vi "load or save device list.vi"(6 "Type":string="Device ", 7 "Mode":u16(ring) items=["Load", "Save"], 10 "selected path":path, 11 "List of devices in":T1 {"List of locations"."Position"."Position Y" format="%#.3f"; "List of locations"."Position"."Position X" format="%#.3f"}) -> (2 "file path out":path, 3 "List of devices out":T1 {"List of locations"."Position"."Position Y" format="%#.3f"; "List of locations"."Position"."Position X" format="%#.3f"})   [LabVIEW 2017]
uses:
  device_list.ctl
  device.ctl
  location.ctl
  <vilib>/Utility/config.llb/Read Key (String).vi
  <vilib>/Utility/config.llb/Write Key (String).vi
  <vilib>/regexp/Match Regular Expression.xnode
  <vilib>/Utility/config.llb/NI_LVConfig.lvlib
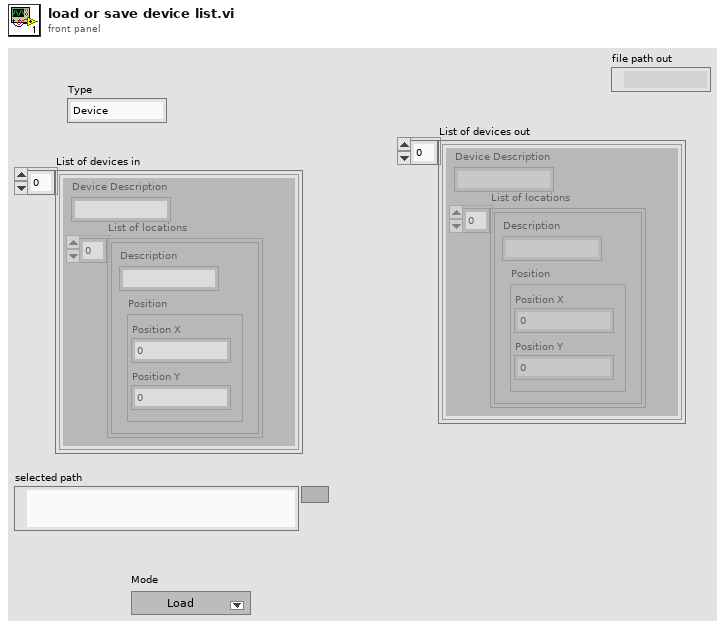
[diagram p1: front panel]
types:
  T1 = typedef "device_list.ctl" = T2[]
  T2 = typedef "device.ctl" = cluster{"List of locations":T3[], "Device Description":string}
  T3 = typedef "location.ctl" = cluster{"Description":string, "Position":cluster{"Position X":dbl, "Position Y":dbl}}
  T4 = typedef "NI_LVConfig.lvlib/Config Data RefNum.ctl" = refnum<k1>
  T5 = cluster{"array type (2D Dbl)[0]":dbl, "array type (2D Dbl)[1]":dbl}
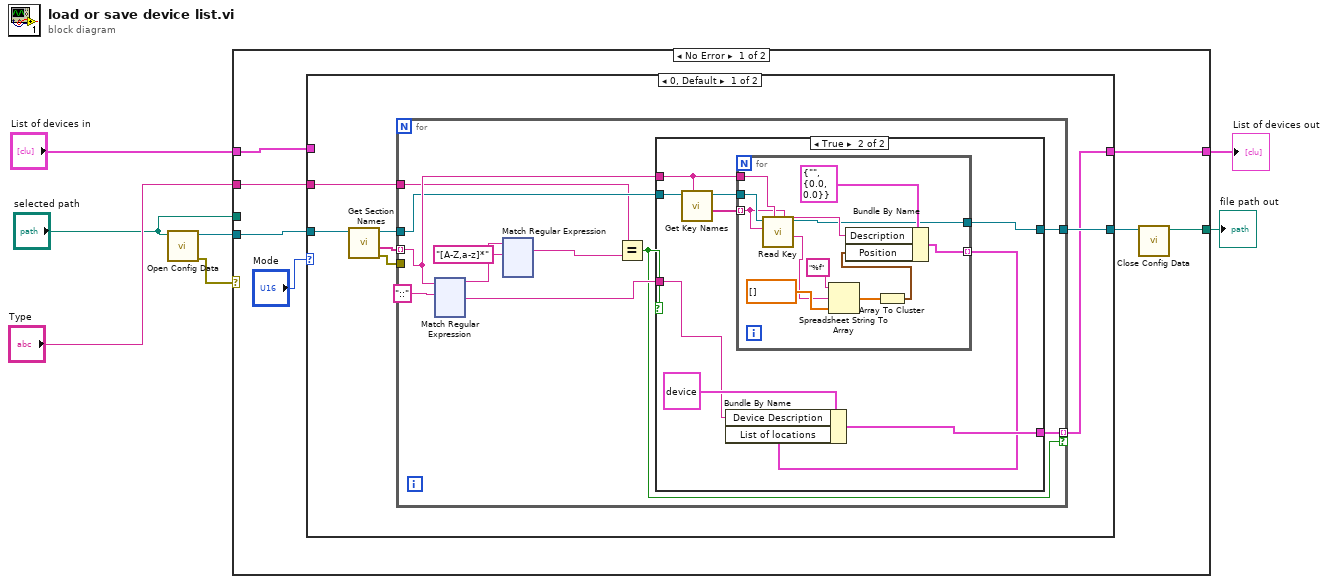
[diagram p0: block diagram]
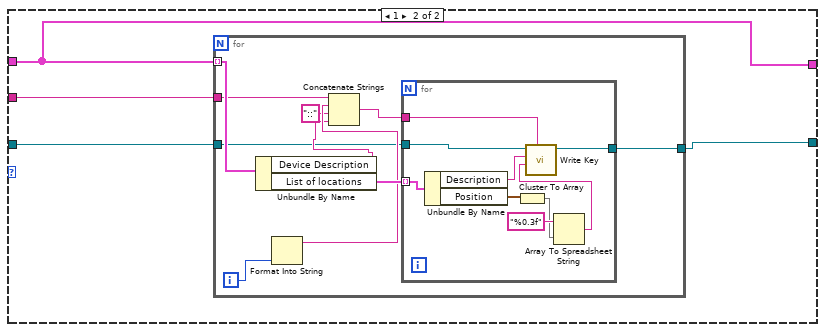
[diagram p3: hidden frame]
diagram:
  n1 = call <vilib>:"Open Config Data.vi"("configuration file path"="selected path") -> ("error out"=w4:errorcluster, "refnum"=w7:T4)  [unwired: 8 in, 1 out]
  n2 = case shown="No Error" w4 {
    tunnel: w7 -> [w14 _]
    tunnel: "List of devices in" -> [w13 w306]
    tunnel: [w10 w306] -> w6
    tunnel: "Type" -> [w9 _]
    tunnel: [w8 w305] -> w2
    tunnel: "selected path" -> [_ w305]
    frame No Error {
      n3 = case shown="0, Default" "Mode" {
        tunnel: w14 -> [w21 w285]
        tunnel: w13 -> [_ w283]
        tunnel: [w18 w284] -> w11
        tunnel: [w17 w283] -> w10
        tunnel: w9 -> [w15 w282]
        frame 0, Default {
          n4 = call <vilib>:"Get Section Names.vi"("refnum"=w21) -> ("error out"=w16:errorcluster, "section names"=w20:string[], "refnum out"=w19:T4)  [unwired: 8 in]
          n5 = for {
            tunnel: w20 -> [w31] mode=indexing
            tunnel: w19 -> [w28]
            tunnel: [w30] -> w18
            tunnel: [w29] -> w17 mode=indexing if=w26
            tunnel: w16 -> [_]
            tunnel: w15 -> [w23]
            n6 = xnode "Match Regular Expression"("input string"=w31, "regular expression"="::") -> ("before match"=w25:string, "after match"=w32:string)  [unwired: 4 in, 3 out]
            n7 = xnode "Match Regular Expression"("input string"=w25, "regular expression"="[A-Z,a-z]*") -> ("whole match"=w22:string)  [unwired: 4 in, 4 out]
            n8 = Equal?(x=w23, y=w22) -> (x = y?=w26:bool)
            n9 = case shown="True" w26 {
              tunnel: w32 -> [_ w154]
              tunnel: w31 -> [_ w152]
              tunnel: [w147 w151] -> w30
              tunnel: [_ w150] -> w29
              tunnel: w28 -> [w147 w149]
              frame False {
              }
              frame True {
                n10 = call <vilib>:"Get Key Names.vi"("section"=w152, "refnum"=w149) -> ("key names"=w156:string[], "refnum out"=w153:T4)  [unwired: 6 in, 2 out]
                n11 = for {
                  tunnel: w156 -> [w162] mode=indexing
                  tunnel: w153 -> [w163]
                  tunnel: w152 -> [w164]
                  tunnel: [w161] -> w151
                  tunnel: [w160] -> w148 mode=indexing
                  n12 = call-poly <vilib>:"Read Key.vi"("section"=w164, "key"=w162, "refnum"=w163) -> ("value"=w158:string, "refnum out"=w161:T4)  [unwired: 5 in, 2 out]
                  n13 = Spreadsheet String To Array(format string="%f", spreadsheet string=w158, array type (2D Dbl)=dbl[] []) -> (array=w165:dbl[])  [unwired: 1 in]
                  n14 = Array To Cluster(array=w165) -> (cluster=w157:T5)
                  n15 = Bundle By Name(cluster=T3 {"Description"="", "Position"={"Position X"=0.0, "Position Y"=0.0}} ("Location"), "Description"=w162, "Position"=w157) -> (w160:T3)
                }
                n16 = Bundle By Name(cluster=T2 {"List of locations"=[{"Description"="Input", "Position"={"Position X"=0.0, "Position Y"=0.0}}, {"Description"="MZI", "Position"={"Position X"=0.0, "Position Y"=10.0}}, {"Description"="Fluid Pool", "Position"={"Position X"=0.0, "Position Y"=20.0}}, {"Description"="Output", "Position"={"Position X"=0.0, "Position Y"=30.0}}], "Device Description"="Default"} ("Defualt Device"), "Device Description"=w154, "List of locations"=w148) -> (w150:T2)
              }
            }
          }
        }
        frame 1 {
          n17 = for {
            tunnel: w283 -> [w295] mode=indexing
            tunnel: w285 -> [w289]
            tunnel: [w288] -> w284
            tunnel: w282 -> [w286]
            i -> [w292]
            n18 = Unbundle By Name(w295) -> ("Device Description"=w290:string, "List of locations"=w294:T3[])
            n19 = Format Into String(w292) -> (resulting string=w291:string)  [unwired: 3 in, 1 out]
            n20 = Concatenate Strings(w286, w291, "::" ("string"), w290) -> (w293:string)
            n21 = for {
              tunnel: w294 -> [w304] mode=indexing
              tunnel: w293 -> [w296]
              tunnel: [w300] -> w288
              tunnel: w289 -> [w297]
              n22 = Unbundle By Name(w304) -> ("Description"=w303:string, "Position"=w302:cluster{"Position X":dbl, "Position Y":dbl})
              n23 = Cluster To Array(cluster=w302) -> (array=w299:dbl[])
              n24 = Array To Spreadsheet String(array=w299, 3:"%0.3f" ("format string")) -> (spreadsheet string=w298:string)  [unwired: 1 in]
              n25 = call-poly <vilib>:"Write Key.vi"("section"=w296, "value"=w298, "key"=w303, "refnum"=w297) -> ("refnum out"=w300:T4)  [unwired: 5 in, 2 out]
            }
          }
        }
      }
      n26 = call <vilib>:"Close Config Data.vi"("refnum"=w11) -> ("file path"=w8:path)  [unwired: 9 in, 1 out]
    }
    frame Error {
    }
  }
  "List of devices out" <- w6
  "file path out" <- w2
